vi "Pick MB port.vi"() -> ()   [LabVIEW 2019]
uses:
  MB Director.ctl
panel:
  in  "Cancel Button":bool
  in  "OK Button":bool
  in  "Modbus Port":refnum<visa-resource-name>
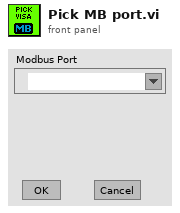
[diagram p1: front panel]
types:
  T1 = typedef "MB Director.ctl" = enum16{"Config MB Port", "Run MB", "Get MB Port", "Quit MB"}
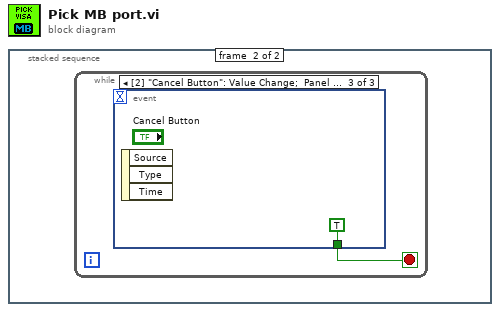
[diagram p0: block diagram]
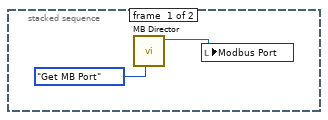
[diagram p2: hidden frame]
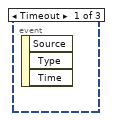
[diagram p3: hidden frame]
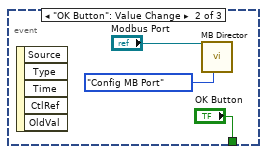
[diagram p4: hidden frame]
diagram:
  n1 = stacked-sequence {
    frame #0 {
      n2 = call "MB Director.vi"("MB Director"=MB_Director."Get MB Port") -> ("MB Port out"=w1:refnum<visa-resource-name>)  [unwired: 9 in, 1 out]
      n3 = local write "Modbus Port"(w1) -> ()
    }
    frame #1 {
      n4 = while {
        stop <- w3 stop-if-true
        n5 = event shown="[2] \"Cancel Button\": Value Change;  Panel Close" {
          selector: _ -> [_ _ _]
          dyn-events: _ -> [_ _ _]
          timeout: _ -> [_ _ _]
          tunnel: [_ "OK Button" TRUE ("OK Button")] -> w3
          event Timeout {
            n6 = event-data() -> ()  [unwired: 1 in, 3 out]
          }
          event "OK Button": Value Change {
            n7 = event-data() -> ()  [unwired: 1 in, 5 out]
            n8 = call "MB Director.vi"("MB Director"=MB_Director."Config MB Port", "MB Port in"="Modbus Port") -> ()  [unwired: 8 in, 2 out]
          }
          event "Cancel Button": Value Change; Panel Close {
            n9 = event-data() -> ()  [unwired: 1 in, 3 out]
          }
        }
      }
    }
  }
